vi "Get Valid Properties.vi"(8 "error in (no error)":errorcluster, 11 "Channel in":refnum<class "Channel.lvclass">) -> (0 "error out":errorcluster, 2 "Properties":string[](array[string]), 3 "Channel out":refnum<class "Channel.lvclass">)   [LabVIEW 2015, in "Channel.lvclass"]
uses:
  Channel.lvclass
  Channel.lvclass/Channel.ctl
  Modulations/AM/AM.lvclass
  Waveforms/Waveform/Waveform.lvclass
  Gate/Gate.lvclass
  Level/Level.lvclass
  Filter/Filter.lvclass
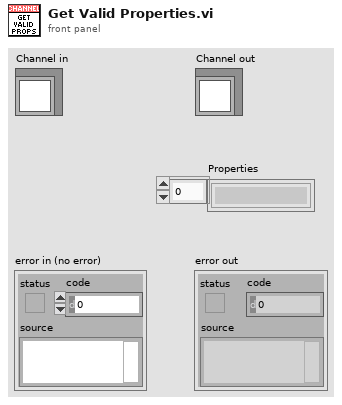
[diagram p1: front panel]
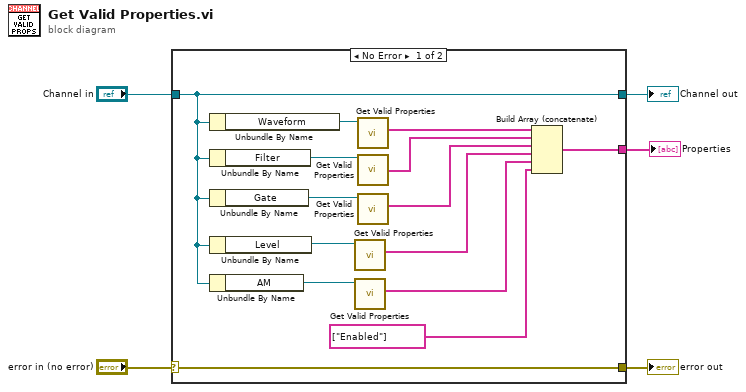
[diagram p0: block diagram]
diagram:
  n1 = case shown="No Error" "error in (no error)" {
    selector: "error in (no error)" -> [w19 w21]
    tunnel: [w19 w21] -> w4
    tunnel: [w8 w20] -> w2
    tunnel: "Channel in" -> [w8 w20]
    tunnel: [w17 _] -> w1
    frame No Error {
      n2 = Unbundle By Name(w8) -> ("Waveform"=w16:refnum<class "Waveform.lvclass">)
      n3 = Unbundle By Name(w8) -> ("Filter"=w7:refnum<class "Filter.lvclass">)
      n4 = Unbundle By Name(w8) -> ("Gate"=w18:refnum<class "Gate.lvclass">)
      n5 = Unbundle By Name(w8) -> ("Level"=w14:refnum<class "Level.lvclass">)
      n6 = Unbundle By Name(w8) -> ("AM"=w11:refnum<class "AM.lvclass">)
      n7 = call "Get Valid Properties.vi"("Level in"=w14) -> ("Properties"=w13:string[])  [unwired: 8 in, 2 out]
      n8 = call-dynamic "Get Valid Properties.vi"("AM in"=w11) -> ("Properties"=w12:string[])  [unwired: 8 in, 2 out]
      n9 = call-dynamic "Get Valid Properties.vi"("Waveform in"=w16) -> ("Properties"=w15:string[])  [unwired: 8 in, 2 out]
      n10 = call "Get Valid Properties.vi"("Filter in"=w7) -> ("Properties"=w9:string[])  [unwired: 12 in, 2 out]
      n11 = call "Get Valid Properties.vi"("Gate in"=w18) -> ("Properties"=w10:string[])  [unwired: 8 in, 2 out]
      n12 = Build Array (concatenate)(w15, w9, w10, w13, w12, string[] ["Enabled"]) -> (w17:string[])
    }
    frame Error {
    }
  }
  "error out" <- w4
  "Channel out" <- w2
  "Properties" <- w1
